vi "Comaptator SubVI v 2.0..vi"(8 "Q":dbl, 11 "P":dbl) -> (0 "P>Q?":bool, 3 "P=Q?":bool)   [LabVIEW 2020]
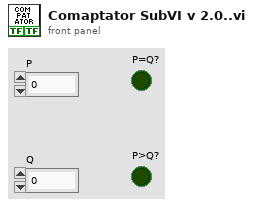
[diagram p1: front panel]
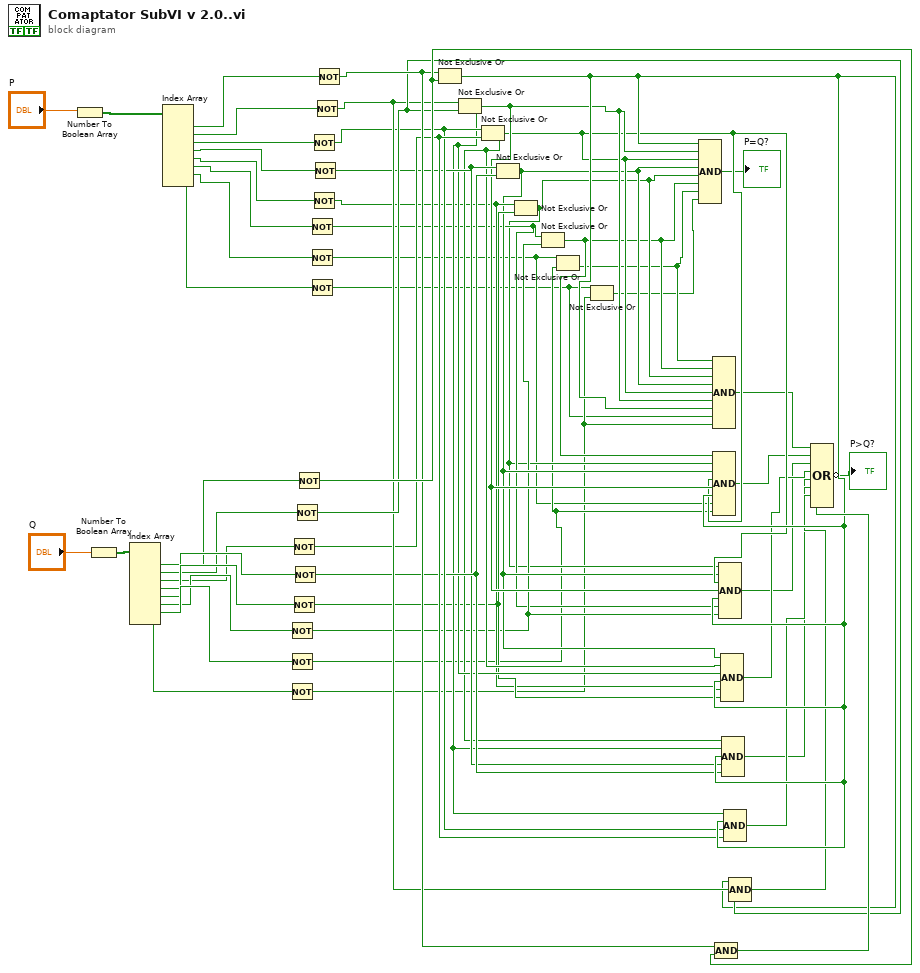
[diagram p0: block diagram]
diagram:
  n1 = Number To Boolean Array(number="P") -> (Boolean array=w3:bool[])
  n2 = Number To Boolean Array(number="Q") -> (Boolean array=w20:bool[])
  n3 = Index Array(array=w20) -> (element #1=w12:bool, element #2=w13:bool, element #3=w14:bool, element #4=w15:bool, element #5=w16:bool, element #6=w17:bool, element #7=w18:bool, element #8=w19:bool)  [unwired: 8 in]
  n4 = Index Array(array=w3) -> (element #1=w4:bool, element #2=w5:bool, element #3=w6:bool, element #4=w7:bool, element #5=w8:bool, element #6=w9:bool, element #7=w10:bool, element #8=w11:bool)  [unwired: 8 in]
  n5 = Not(x=w17) -> (.not. x?=w33:bool)
  n6 = Not(x=w18) -> (.not. x?=w30:bool)
  n7 = Not(x=w19) -> (.not. x?=w26:bool)
  n8 = Not(x=w14) -> (.not. x?=w47:bool)
  n9 = Not(x=w16) -> (.not. x?=w39:bool)
  n10 = Not(x=w15) -> (.not. x?=w45:bool)
  n11 = Not(x=w13) -> (.not. x?=w51:bool)
  n12 = Not(x=w12) -> (.not. x?=w54:bool)
  n13 = Not(x=w9) -> (.not. x?=w32:bool)
  n14 = Not(x=w10) -> (.not. x?=w29:bool)
  n15 = Not(x=w11) -> (.not. x?=w25:bool)
  n16 = Not(x=w6) -> (.not. x?=w46:bool)
  n17 = Not(x=w8) -> (.not. x?=w38:bool)
  n18 = Not(x=w7) -> (.not. x?=w44:bool)
  n19 = Not(x=w5) -> (.not. x?=w50:bool)
  n20 = Not(x=w4) -> (.not. x?=w53:bool)
  n21 = Not Exclusive Or(1:w54, 2:w53) -> (0:w49:bool)
  n22 = Not Exclusive Or(1:w51, 2:w50) -> (0:w43:bool)
  n23 = Not Exclusive Or(1:w47, 2:w46) -> (0:w41:bool)
  n24 = Not Exclusive Or(1:w45, 2:w44) -> (0:w37:bool)
  n25 = Not Exclusive Or(1:w39, 2:w38) -> (0:w31:bool)
  n26 = Not Exclusive Or(1:w33, 2:w32) -> (0:w28:bool)
  n27 = Not Exclusive Or(1:w30, 2:w29) -> (0:w27:bool)
  n28 = Not Exclusive Or(1:w26, 2:w25) -> (0:w21:bool)
  n29 = Compound Arithmetic op=AND(w49, w43, w41, w37, w31, w28, w27, w21) -> (→"P=Q?":bool)
  n30 = Compound Arithmetic op=AND(w27, w28, w31, w37, w41, w43, w49, w25, w26) -> (w24:bool)
  n31 = Compound Arithmetic op=AND(w28, w31, w37, w41, w43, w49, w29, w30) -> (w35:bool)
  n32 = Compound Arithmetic op=AND(w53, w54) -> (w52:bool)
  n33 = Compound Arithmetic op=AND(w31, w37, w41, w43, w49, w32, w33) -> (w34:bool)
  n34 = Compound Arithmetic op=AND(w37, w41, w43, w49, w38, w39) -> (w36:bool)
  n35 = Compound Arithmetic op=AND(w41, w43, w49, w44, w45) -> (w40:bool)
  n36 = Compound Arithmetic op=AND(w43, w49, w46, w47) -> (w42:bool)
  n37 = Compound Arithmetic op=AND(w49, w50, w51) -> (w48:bool)
  n38 = Compound Arithmetic op=OR(w24, w35, w34, w36, w40, w42, w48, w52) -> (invert →"P>Q?":bool)
